vi "fpga.vi"() -> ()   [LabVIEW 2012]
uses:
  <vilib>/eio/EIONode/EIONode.xnode
  <vilib>/rvi/eio/common/nirviEmuTemplateMethod_errors.vi
panel:
  in  "PWM 15":u32=1500
  in  "PWM 31":u32=1500
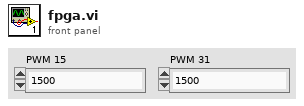
[diagram p1: front panel]
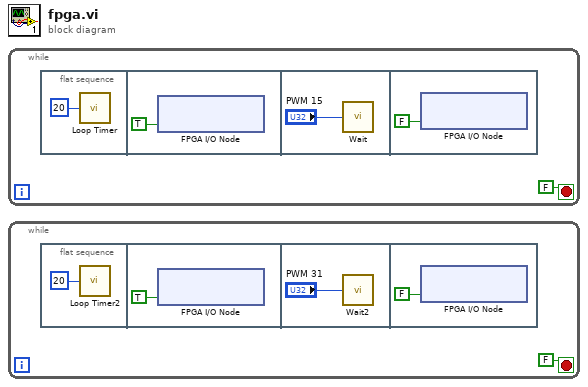
[diagram p0: block diagram]
diagram:
  n1 = while {
    stop <- FALSE stop-if-true
    n2 = flat-sequence {
      frame #0 {
        n3 = call "Loop Timer"("Count(mSec)"=u8 20) -> ()  [unwired: 1 out]
      }
      frame #1 {
        n4 = xnode "FPGA I/O Node"("RMC/DIO15"=TRUE) -> ()  [unwired: 1 in, 1 out]
      }
      frame #2 {
        n5 = call "Wait"("Count(uSec)"="PWM 15") -> ()  [unwired: 1 out]
      }
      frame #3 {
        n6 = xnode "FPGA I/O Node"("RMC/DIO15"=FALSE) -> ()  [unwired: 1 in, 1 out]
      }
    }
  }
  n7 = while {
    stop <- FALSE stop-if-true
    n8 = flat-sequence {
      frame #0 {
        n9 = call "Loop Timer2"("Count(mSec)"=u8 20) -> ()  [unwired: 1 out]
      }
      frame #1 {
        n10 = xnode "FPGA I/O Node"("RMC/DIO31"=TRUE ("RMC/DIO15")) -> ()  [unwired: 1 in, 1 out]
      }
      frame #2 {
        n11 = call "Wait2"("Count(uSec)"="PWM 31") -> ()  [unwired: 1 out]
      }
      frame #3 {
        n12 = xnode "FPGA I/O Node"("RMC/DIO31"=FALSE ("RMC/DIO15")) -> ()  [unwired: 1 in, 1 out]
      }
    }
  }
